vi "set view class name.vi"(8 "error in":errorcluster, 10 "view class":string, 11 "CEF_Configuration in":refnum<class "CEF_serializable configuration.lvclass">) -> (0 "error out":errorcluster, 3 "CEF_Configuration out":refnum<class "CEF_serializable configuration.lvclass">)   [LabVIEW 2025, in "CEF.lvlib" / "CEF_serializable configuration.lvclass"]
doc: "Copyright 2017 National Instruments Corporation\n\nLicensed under the Apache License, Version 2.0 (the \"License\"); you may not use this file except in compliance with the License. You may obtain a copy of the License at http://www.apache.org/licenses/LICENSE-2.0\nUnless required by applicable law or agreed to in writing, software distributed under the License is distributed on an \"AS IS\" BASIS, WITHOUT WARRANTIES OR CONDITIONS OF ANY KIND, either express or implied. See the License for the specific language governing permissions and limitations under the License."
uses:
  CEF_serializable configuration.lvclass
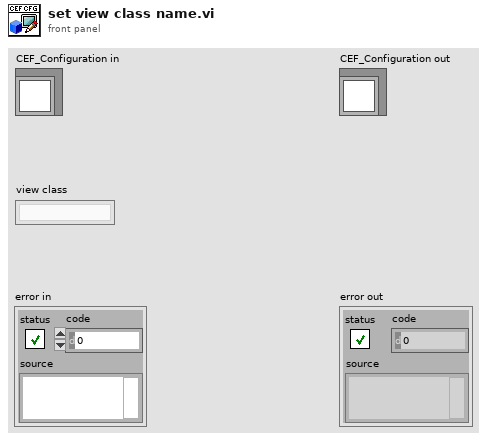
[diagram p1: front panel]
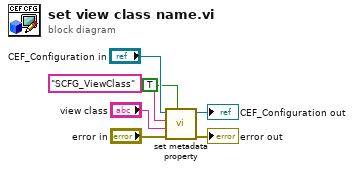
[diagram p0: block diagram]
diagram:
  n1 = call "set metadata property.vi"("overwrite?"=TRUE, "error in"="error in", "value"="view class", "key"="SCFG_ViewClass", "CEF_Configuration in"="CEF_Configuration in") -> ("error out"=→"error out":errorcluster, "CEF_Configuration out"=→"CEF_Configuration out":refnum<class "CEF_serializable configuration.lvclass">)  [unwired: 5 in]
